vi "SwerveModuleState_Get.vi"(11 "Desired State":T1={"Speed"=0.0, "Angle"={"VALUE"=0.0, "COS"=1.0, "SIN"=0.0}} {"Angle"."SIN" format="%13.4f"; "Angle"."COS" format="%13.4f"; "Angle"."VALUE" format="%13.4f"}) -> (1 "Angle RADIANS":dbl, 3 "Speed M/S":dbl)   [LabVIEW 2019, in "Trajectory_Library.lvlib"]
doc: "Get the individual speed (meters/sec) and angle (radians) components of the Module State data cluster.\n\nParmeters:\n - Module State\n\nReturns:\n - Speed -- Module speed (Meters/Sec)\n - Angle -- Module angle (Radians)"
uses:
  Trajectory_Library.lvlib
  TypeDef/SWERVE_DRIVE_MODULE_STATE.ctl
  TypeDef/ROTATION2D.ctl
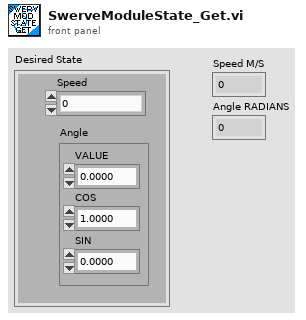
[diagram p1: front panel]
types:
  T1 = typedef "Trajectory_Library.lvlib/SWERVE_DRIVE_MODULE_STATE.ctl" = cluster{"Speed":dbl, "Angle":T2}
  T2 = typedef "Trajectory_Library.lvlib/ROTATION2D.ctl" = cluster{"VALUE":dbl, "COS":dbl, "SIN":dbl}
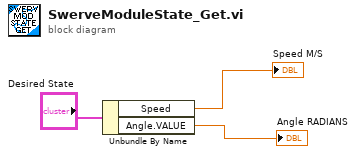
[diagram p0: block diagram]
diagram:
  n1 = Unbundle By Name("Desired State") -> ("Speed"=→"Speed M/S":dbl, "Angle.VALUE"=→"Angle RADIANS":dbl)
